vi "Atividade 1.vi"() -> ()   [LabVIEW 2010]
uses:
  <vilib>/Utility/error.llb/DialogType.ctl
  <vilib>/_DAQmxBase/Internals/DAQmxBase Read (Analog 2D DBL NChan NSamp).vi
panel:
  in  "Samples per Channel":i32=1000
  in  "DAQmxBase Task":refnum<k21>="ai finite dig trig"
  out "Seno/consseno":dbl
  out "Seno?":bool
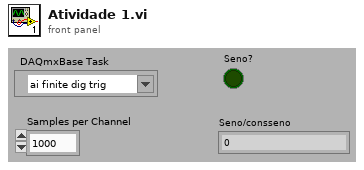
[diagram p1: front panel]
types:
  T1 = typedef "DialogType.ctl" = u16
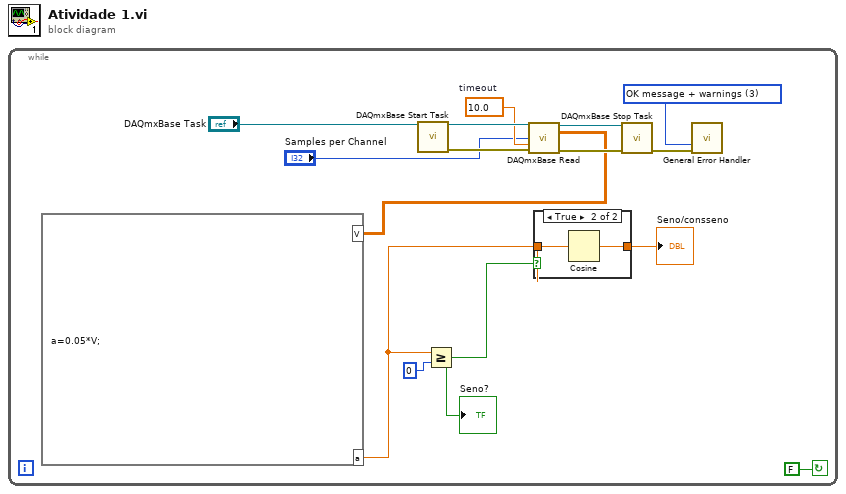
[diagram p0: block diagram]
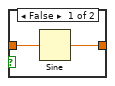
[diagram p2: hidden frame]
diagram:
  n1 = while {
    stop <- FALSE continue-if-true
    w4 = T1 3 items=["no dialog", "OK message", "continue or stop message", "OK message + warnings", "continue/stop + warnings"] ("type of dialog (OK msg:1)")
    w6 = 10.0  # timeout
    n2 = call <vilib>:"DAQmxBase Start Task.vi"("task/channels in"="DAQmxBase Task") -> ("task out"=w8:refnum<k21>, "error out"=w10:errorcluster)  [unwired: 13 in]
    n3 = call-poly <vilib>:"DAQmxBase Read.vi"("task/channels in"=w8, "number of samples per channel"="Samples per Channel", "timeout"=w6, "error in"=w10) -> ("task out"=w7:refnum<k21>, "data"=w1:dbl[][], "error out"=w5:errorcluster)  [unwired: 9 in]
    n4 = formula code="a=0.05*V;"("V"=w1) -> ("a"=w11:dbl)
    n5 = Greater Or Equal?(x=w11, y=0) -> (x >= y?=w13:bool)
    "Seno?" <- w13
    n6 = case shown="True" w13 {
      tunnel: [w17 w19] -> w12
      tunnel: w11 -> [w16 w18]
      frame False {
        n7 = Sine(x=w16) -> (sin(x)=w17:dbl)
      }
      frame True {
        n8 = Cosine(x=w18) -> (cos(x)=w19:dbl)
      }
    }
    "Seno/consseno" <- w12
    n9 = call <vilib>:"DAQmxBase Stop Task.vi"("task/channels in"=w7, "error in"=w5) -> ("error out"=w9:errorcluster)  [unwired: 12 in, 1 out]
    n10 = call <vilib>:"General Error Handler.vi"("type of dialog (OK msg:1)"=w4, "error in (no error)"=w9) -> ()  [unwired: 9 in, 5 out]
  }
